vi "Read TagY.vi"(0 "Tag in":refnum<class "Tag.lvclass">, 1 "error in (no error)":errorcluster) -> (2 "Tag out":refnum<class "Tag.lvclass">, 3 "RealTagY":dbl, 4 "error out":errorcluster)   [LabVIEW 2014, in "Tag.lvclass"]
uses:
  Tag.lvclass
  Tag.lvclass/Tag.ctl
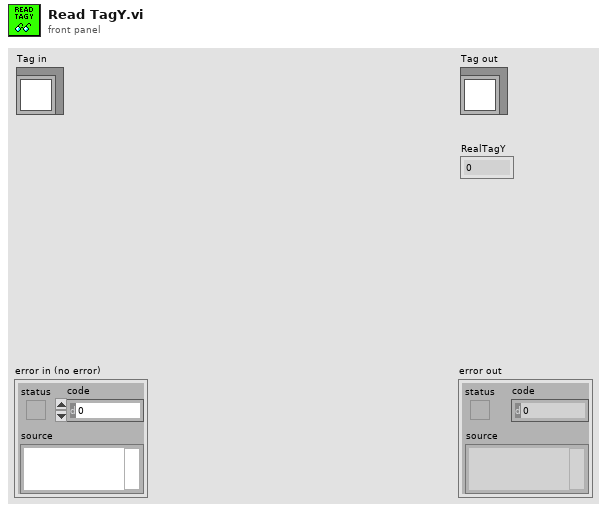
[diagram p1: front panel]
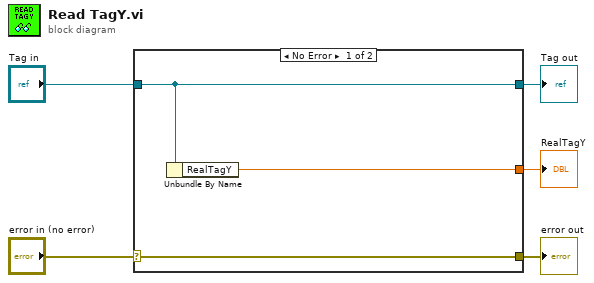
[diagram p0: block diagram]
diagram:
  n1 = case shown="No Error" "error in (no error)" {
    selector: "error in (no error)" -> [w8 w9]
    tunnel: [w8 w9] -> w4
    tunnel: [w7 w10] -> w2
    tunnel: "Tag in" -> [w7 w10]
    tunnel: [w6 _] -> w1
    frame No Error {
      n2 = Unbundle By Name(w7) -> ("RealTagY"=w6:dbl)
    }
    frame Error {
    }
  }
  "error out" <- w4
  "Tag out" <- w2
  "RealTagY" <- w1
